vi "K2400_write&read.vi"(2 "error in (no error)":errorcluster, 3 "Command":string, 4 "VISA Resource Name":refnum<visa-resource-name>) -> (0 "error out":errorcluster, 1 "Read":string)   [LabVIEW 2011]
panel:
  out "VISA resource name out":refnum<visa-resource-name>
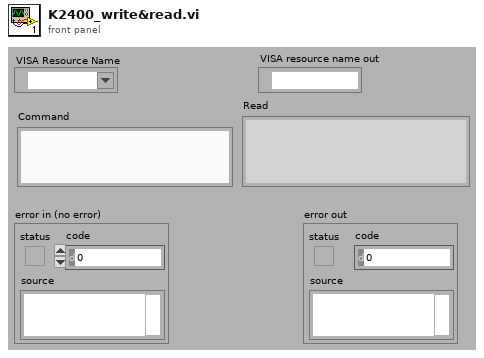
[diagram p1: front panel]
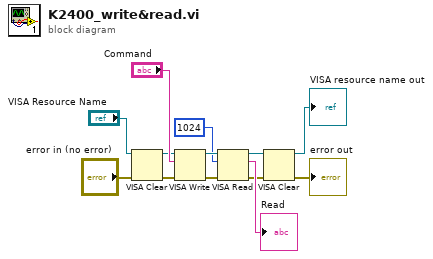
[diagram p0: block diagram]
diagram:
  n1 = VISA Clear(VISA resource name="VISA Resource Name", error in (no error)="error in (no error)") -> (VISA resource name out=w1:refnum<visa-resource-name>, error out=w3:errorcluster)
  n2 = VISA Write(VISA resource name=w1, write buffer="Command", error in (no error)=w3) -> (VISA resource name out=w12:refnum<visa-resource-name>, error out=w10:errorcluster)  [unwired: 1 out]
  n3 = VISA Read(VISA resource name=w12, byte count=1024, error in (no error)=w10) -> (VISA resource name out=w6:refnum<visa-resource-name>, read buffer=→"Read":string, error out=w8:errorcluster)  [unwired: 1 out]
  n4 = VISA Clear(VISA resource name=w6, error in (no error)=w8) -> (VISA resource name out=→"VISA resource name out":refnum<visa-resource-name>, error out=→"error out":errorcluster)
